vi "Example 1.vi"(8 "error in":errorcluster, 10 "base path":path) -> (0 "error out":errorcluster, 2 "JMP log":string)   [LabVIEW 2019]
uses:
  <instrlib>/LV_JMP_bridge/JMP Automation.lvlib
  <vilib>/numeric/Random Number (Range) DBL.vi
  <instrlib>/LV_JMP_bridge/DataTable/Add DataTable Variable (string).vi
  <instrlib>/LV_JMP_bridge/DataTable/Add DataTable Variable (double).vi
  <instrlib>/LV_JMP_bridge/DataTable/Fill DataTable (double array).vi
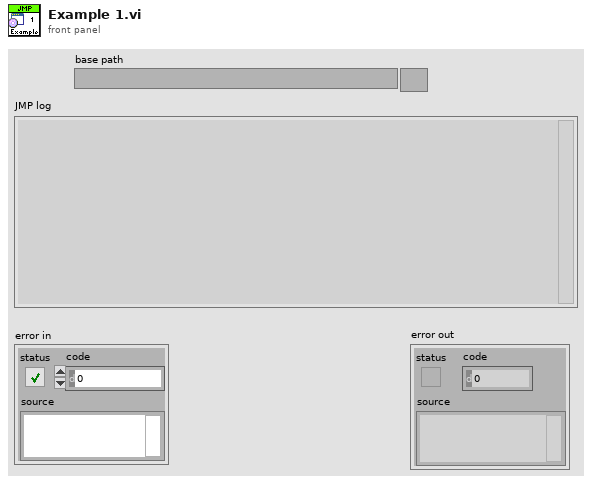
[diagram p1: front panel]
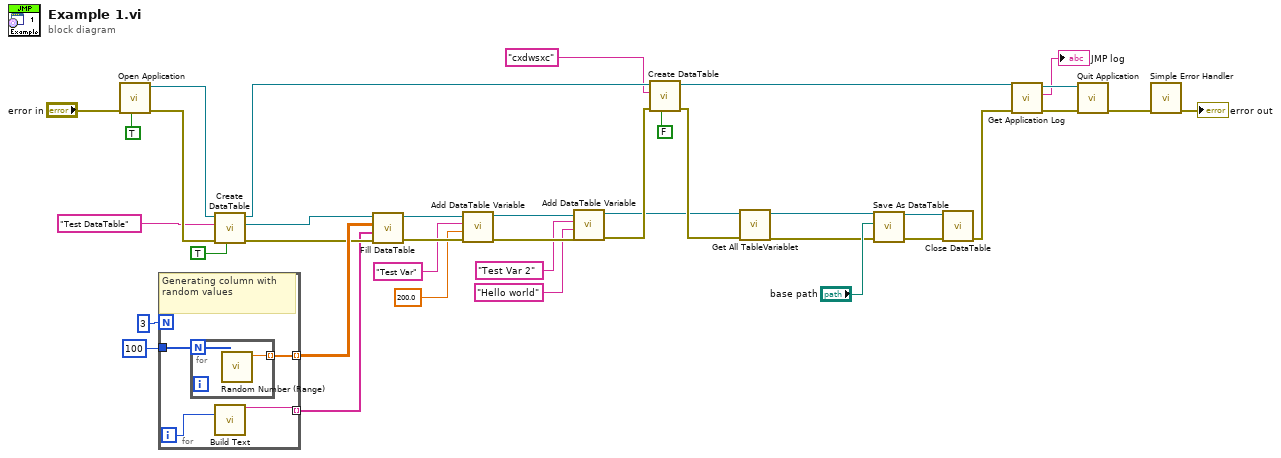
[diagram p0: block diagram]
diagram:
  n1 = call <instrlib>:"Open Application.vi"("visible (false)"=TRUE ("visible"), "error in (no error)"="error in") -> ("error out"=w38:errorcluster, "JMP application"=w19:refnum<k7>)  [unwired: 8 in]
  n2 = for {
    N: 3 -> [_]
    tunnel: [w42] -> w36 mode=indexing
    tunnel: 100 -> [w41]
    tunnel: [w39] -> w20 mode=indexing
    i -> [w40]
    # "Generating column with random values"
    n3 = for {
      N: w41 -> [_]
      tunnel: [w43] -> w42 mode=indexing
      n4 = call-poly <vilib>:"Random Number (Range).vi"() -> ("number"=w43:dbl)  [unwired: 11 in]
    }
    n5 = call "Build Text"("number"=w40) -> ("Result"=w39:string)  [unwired: 13 in, 1 out]
  }
  n6 = call <instrlib>:"Create DataTable.vi"("visible (false)"=TRUE, "error in (no error)"=w38, "table name"="Test DataTable", "JMP application"=w19) -> ("error out"=w32:errorcluster, "new DataTable"=w33:refnum<k7>, "JMP application out"=w16:refnum<k7>)  [unwired: 5 in]
  n7 = call-poly <instrlib>:"Fill DataTable.vi"("error in (no error)"=w32, "columns name"=w20, "columns data"=w36, "JMP DataTable"=w33) -> ("error out"=w17:errorcluster, "JMP DataTable out"=w18:refnum<k7>)  [unwired: 6 in]
  n8 = call-poly <instrlib>:"Add DataTable Variable.vi"("error in (no error)"=w17, "value"=200.0, "name"="Test Var", "JMP DataTable"=w18) -> ("error out"=w4:errorcluster, "JMP data table out"=w3:refnum<k7>)  [unwired: 6 in]
  n9 = call-poly <instrlib>:"Add DataTable Variable.vi"("error in (no error)"=w4, "value"="Hello world", "name"="Test Var 2", "JMP DataTable"=w3) -> ("error out"=w14:errorcluster, "JMP data table out"=w8:refnum<k7>)  [unwired: 6 in]
  n10 = call <instrlib>:"Create DataTable.vi"("visible (false)"=FALSE, "error in (no error)"=w14, "table name"="cxdwsxc", "JMP application"=w16) -> ("error out"=w9:errorcluster, "JMP application out"=w11:refnum<k7>)  [unwired: 5 in, 1 out]
  n11 = call <instrlib>:"Get All TableVariablet.vi"("error in (no error)"=w9, "DataTable"=w8) -> ("error out"=w10:errorcluster, "DataTable out"=w7:refnum<k7>)  [unwired: 8 in]
  n12 = call <instrlib>:"Save As DataTable.vi"("error in (no error)"=w10, "filepath"="base path", "JMP DataTable"=w7) -> ("error out"=w31:errorcluster, "JMP data table out"=w30:refnum<k7>)  [unwired: 7 in]
  n13 = call <instrlib>:"Close DataTable.vi"("error in (no error)"=w31, "JMP DataTable"=w30) -> ("error out"=w27:errorcluster)  [unwired: 9 in]
  n14 = call <instrlib>:"Get Application Log.vi"("error in (no error)"=w27, "JMP application"=w11) -> ("error out"=w28:errorcluster, "JMP log"=→"JMP log":string, "JMP application out"=w29:refnum<k7>)  [unwired: 7 in]
  n15 = call <instrlib>:"Quit Application.vi"("error in (no error)"=w28, "JMP application"=w29) -> ("error out"=w37:errorcluster)  [unwired: 9 in]
  n16 = call <vilib>:"Simple Error Handler.vi"("error in (no error)"=w37) -> ("error out"=→"error out":errorcluster)  [unwired: 4 in, 4 out]
